vi "解析包.vi"(1 "数据包队列名称":refnum<queue>) -> (0 "解析包状态":bool=TRUE)   [LabVIEW 2017]
panel:
  out "取包次数":dbl=43.0
  in  "引导码":string[](array[string])=["boot_message", "boot_arg", "boot_image", "boot_cmdres", "boot_pcap", ""]
  out "当前引导码":string
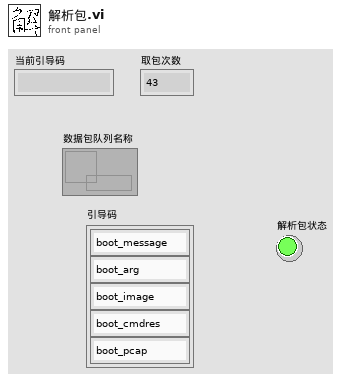
[diagram p1: front panel]
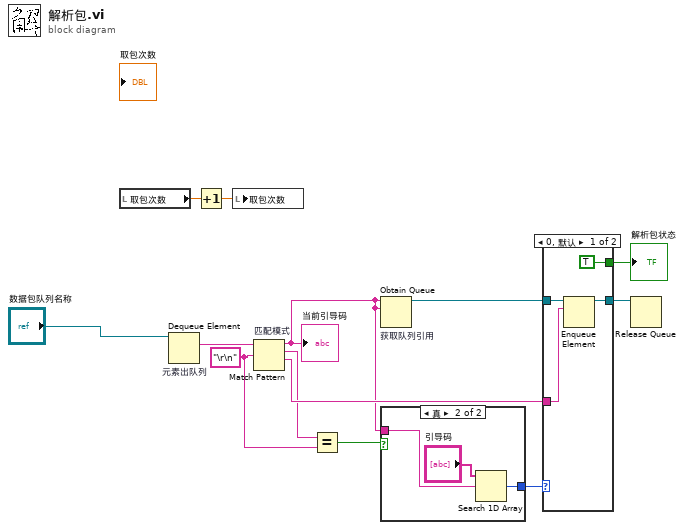
[diagram p0: block diagram]
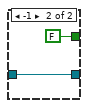
[diagram p2: hidden frame]
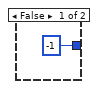
[diagram p3: hidden frame]
diagram:
  w2 = "\r\n" ("正则表达式")
  n1 = local read "取包次数"() -> (w10:dbl)
  n2 = Dequeue Element "元素出队列"(queue="数据包队列名称") -> (element=w12:string)  [unwired: 2 in, 3 out]
  n3 = Increment(x=w10) -> (x+1=w11:dbl)
  n4 = local write "取包次数"(w11) -> ()
  n5 = Match Pattern "匹配模式"(string=w12, regular expression=w2) -> (before substring=w4:string, match substring=w3:string, after substring=w6:string)  [unwired: 1 in, 1 out]
  "当前引导码" <- w4
  n6 = Equal?(x=w3, y=w2) -> (x = y?=w1:bool)
  n7 = Obtain Queue "获取队列引用"(name (unnamed)=w4, element data type=w4) -> (queue out=w5:refnum<queue>)  [unwired: 3 in, 2 out]
  n8 = case shown="真" w1 {
    tunnel: w4 -> [_ w15]
    tunnel: [-1 w17] -> w9
    frame False {
    }
    frame True {
      n9 = Search 1D Array(1D array="引导码", element=w15) -> (index of element=w17:i32)  [unwired: 1 in]
    }
  }
  n10 = case shown="0, 默认" w9 {
    tunnel: w5 -> [w21 w23]
    tunnel: [w20 w23] -> w8
    tunnel: [TRUE ("解析包状态") FALSE ("解析包状态")] -> w7
    tunnel: w6 -> [w18 _]
    frame 0, Default {
      n11 = Enqueue Element(queue=w21, element=w18) -> (queue out=w20:refnum<queue>)  [unwired: 2 in, 2 out]
    }
    frame -1 {
    }
  }
  "解析包状态" <- w7
  n12 = Release Queue(queue=w8) -> ()  [unwired: 2 in, 3 out]
